vi "Noise_Generator.vi"() -> ()   [LabVIEW 2018]
uses:
  Global_Noise.vi
  <vilib>/Analysis/NI_AALBase.lvlib
panel:
  out "Running":bool
  in  "Power":bool
  in  "Initiallize":bool=TRUE
  in  "Samples":i32=1000 min=0
  in  "Seed":i8=-1
  in  "Amplitude":dbl=5.0
  out "Waveform Graph":dbl[](graph)
  # "Noise Generator"
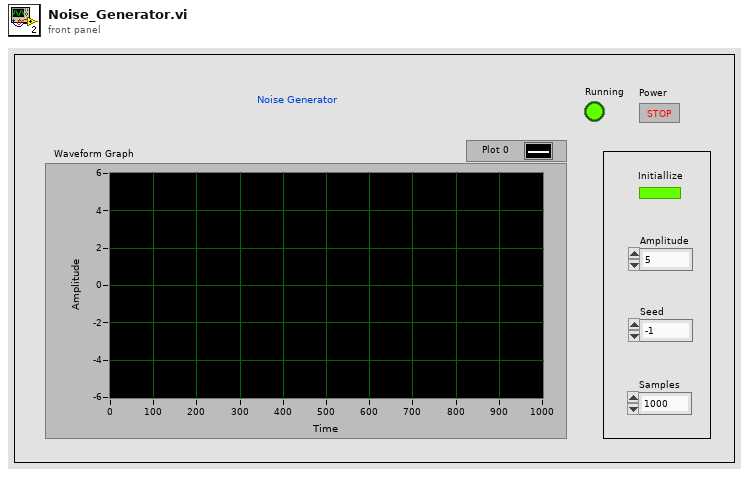
[diagram p1: front panel]
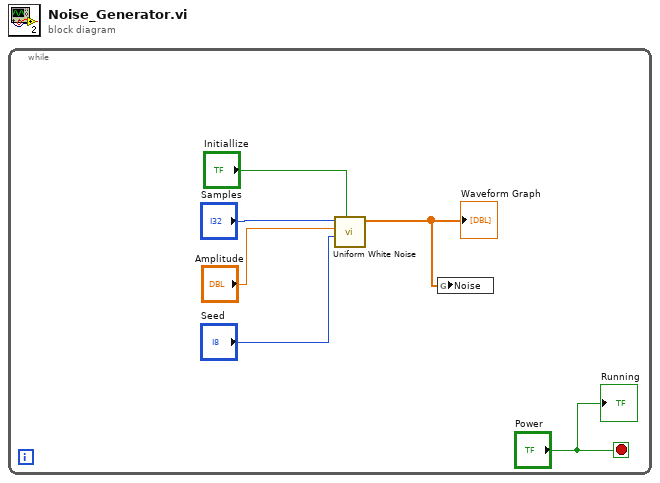
[diagram p0: block diagram]
diagram:
  n1 = while {
    stop <- "Power" stop-if-true
    n2 = call <vilib>:"Uniform White Noise.vi"("initialize?"="Initiallize", "seed"="Seed", "amplitude"="Amplitude", "samples"="Samples") -> ("uniform white noise"=w1:dbl[])  [unwired: 6 in, 1 out]
    "Waveform Graph" <- w1
    n3 = global write "Global_Noise.vi" "Noise"(w1) -> ()
    "Running" <- "Power"
  }
